vi "FW102C Engine.vi"(0 "Notifier Name":string="Not a Name", 11 "COM Port":string[](array[string])) -> ()   [LabVIEW 2016]
uses:
  FW Type Defs/FW Notifier Type.ctl
  FW Type Defs/FW Actions.ctl
  FilterWheel102_win64.dll
panel:
  out "FW ID":string
  out "Current Position":u8
  in  "Get Position":bool
  in  "FW Position":u8
  in  "Quit":bool
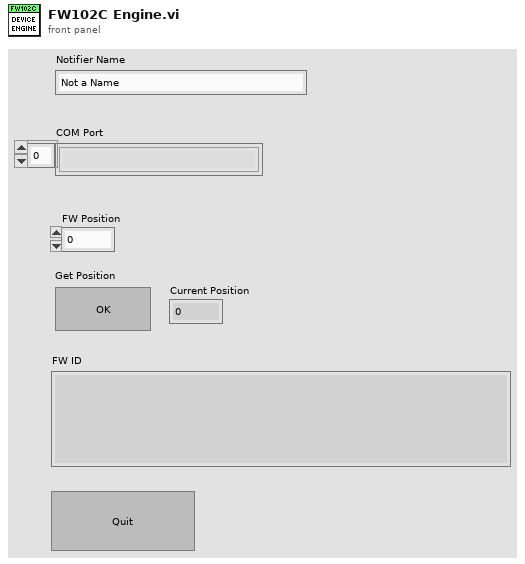
[diagram p1: front panel]
types:
  T1 = typedef "FW Actions.ctl" = enum16{"Set Position", "Get Position", "Get Num Positions", "Set Speed", "Quit"}
  T2 = typedef "FW Notifier Type.ctl" = cluster{"Actions":T1, "Set Position":u8, "Actual Position":u8, "Speed":dbl, "Num Positions":u8, "Received":bool}
  T3 = enum32{"Invalid", "Standard", "Closed", "Hidden", "Minimized", "Maximized"}
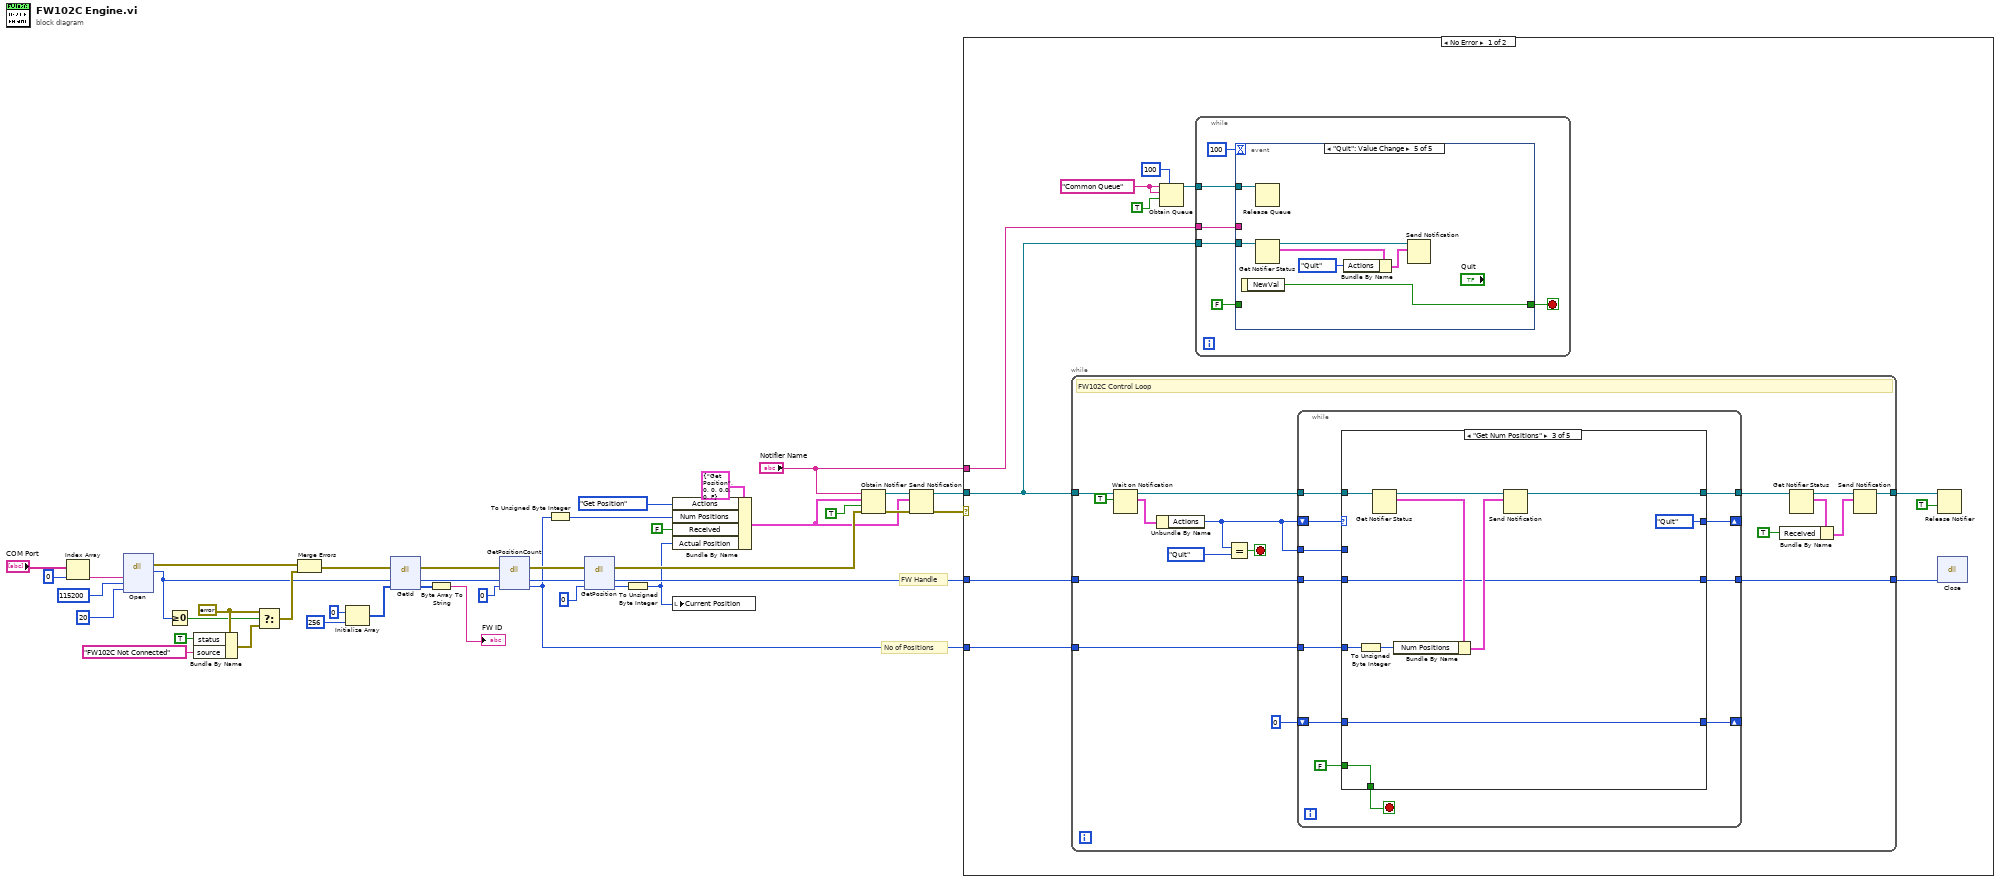
[diagram p0: block diagram]
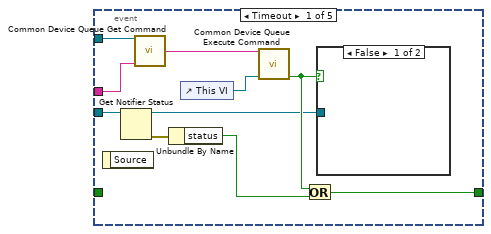
[diagram p2: hidden frame]
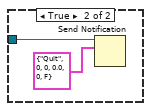
[diagram p3: hidden frame]
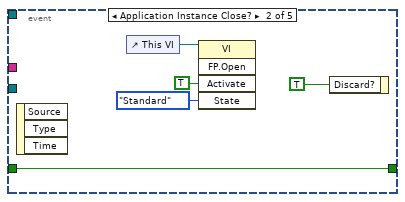
[diagram p4: hidden frame]
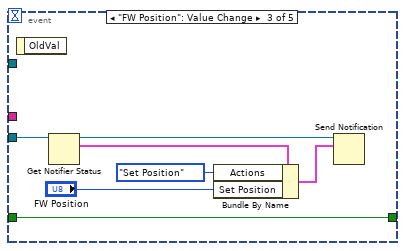
[diagram p5: hidden frame]
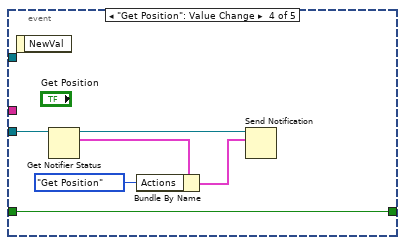
[diagram p6: hidden frame]
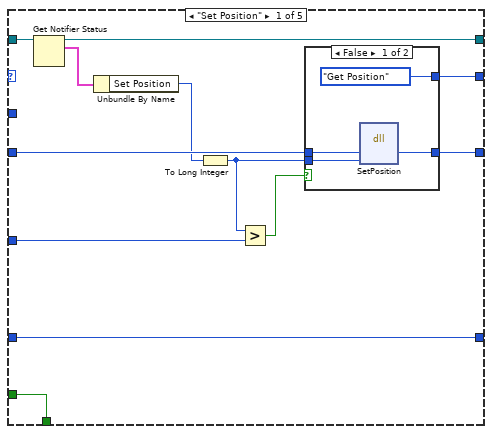
[diagram p7: hidden frame]
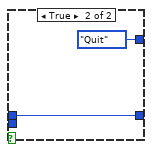
[diagram p8: hidden frame]
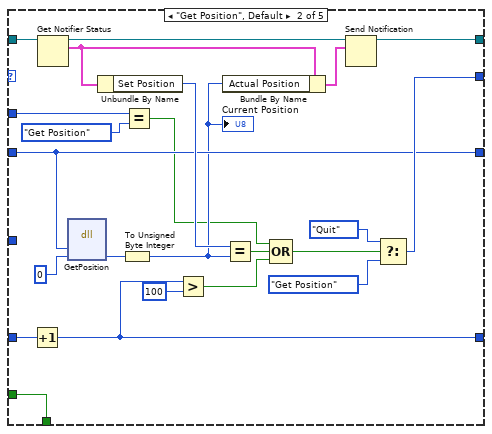
[diagram p9: hidden frame]
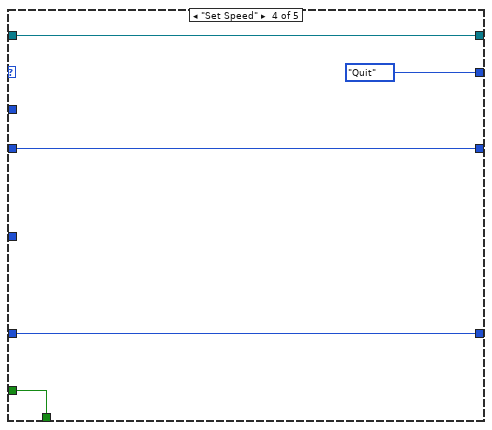
[diagram p10: hidden frame]
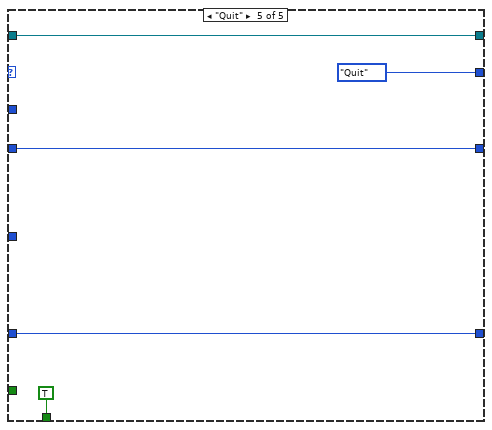
[diagram p11: hidden frame]
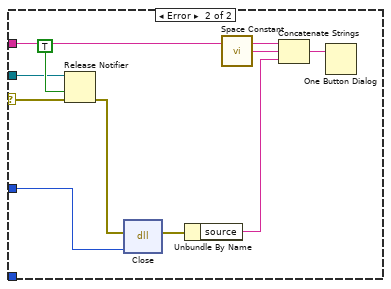
[diagram p12: hidden frame]
diagram:
  w30 = errorcluster {"status"=FALSE, "code"=0, "source"=""} ("error out")
  # "No of Positions"
  # "FW Handle"
  n1 = Index Array(array="COM Port", index=0) -> (element=w31:string)
  n2 = dll-call lib="C:/Users/gs519/Documents/Microscope-Control/Device Library/Filter Wheels/Thorlabs/FW102C/FilterWheel102_win64.dll" fn="Open"("Serial No"=w31, "nBaud"=115200 ("nbaud"), "timeout"=20) -> (error out=w25:errorcluster, "hdl"=w18:i32)  [unwired: 6 in, 1 out]
  n3 = Greater Or Equal To 0?(x=w18) -> (x >= 0?=w26:bool)
  n4 = Bundle By Name(cluster=w30, "status"=TRUE, "source"="FW102C Not Connected") -> (w27:errorcluster)
  n5 = Select(t=w30, s=w26, f=w27) -> (s? t:f=w24:errorcluster)
  n6 = Merge Errors(w25, w24) -> (w17:errorcluster)
  n7 = Initialize Array(u8 0 ("element"), 256 ("dimension size")) -> (w21:u8[])
  n8 = dll-call lib="C:/Users/gs519/Documents/Microscope-Control/Device Library/Filter Wheels/Thorlabs/FW102C/FilterWheel102_win64.dll" fn="GetId"(error in=w17, "hdl"=w18, "id"=w21) -> (error out=w15:errorcluster, "hdl"=w14:i32, "id"=w19:u8[])  [unwired: 3 in, 1 out]
  n9 = Byte Array To String(unsigned byte array=w19) -> (string=→"FW ID":string)
  n10 = dll-call lib="C:/Users/gs519/Documents/Microscope-Control/Device Library/Filter Wheels/Thorlabs/FW102C/FilterWheel102_win64.dll" fn="GetPositionCount" label="GetCount"(error in=w15, "hdl"=w14, "position count"=0) -> (error out=w12:errorcluster, "hdl"=w11:i32, "position count"=w2:i32)  [unwired: 3 in, 1 out]
  n11 = To Unsigned Byte Integer(number=w2) -> (unsigned 8bit integer=w1:u8)
  n12 = dll-call lib="C:/Users/gs519/Documents/Microscope-Control/Device Library/Filter Wheels/Thorlabs/FW102C/FilterWheel102_win64.dll" fn="GetPosition"(error in=w12, "hdl"=w11, "position"=0) -> (error out=w10:errorcluster, "hdl"=w9:i32, "position"=w5:i32)  [unwired: 3 in, 1 out]
  n13 = To Unsigned Byte Integer(number=w5) -> (unsigned 8bit integer=w3:u8)
  n14 = Bundle By Name(cluster=T2 {"Actions"=enum."Get Position", "Set Position"=0, "Actual Position"=0, "Speed"=0.0, "Num Positions"=0, "Received"=FALSE} ("Note Type"), "Actions"=FW_Actions."Get Position", "Num Positions"=w1, "Received"=FALSE ("Received?"), "Actual Position"=w3) -> (w4:T2)
  n15 = local write "Current Position"(w3) -> ()
  n16 = Obtain Notifier(name (unnamed)="Notifier Name", notification data type=w4, create if not found? (T)=TRUE, error in (no error)=w10) -> (notifier out=w40:refnum<notifier>, error out=w39:errorcluster)  [unwired: 1 out]
  n17 = Send Notification(notification=w4, notifier=w40, error in (no error)=w39) -> (notifier out=w38:refnum<notifier>, error out=w37:errorcluster)
  n18 = case shown="No Error" w37 {
    selector: w37 -> [_ w194]
    tunnel: w38 -> [w50 w195]
    tunnel: "Notifier Name" -> [w49 w193]
    tunnel: w9 -> [w44 w190]
    tunnel: w2 -> [w42 _]
    frame No Error {
      w48 = "Common Queue" ("Unique Notifier Name")
      n19 = while {
        tunnel: w50 -> [w106]
        tunnel: [w107] -> w51
        tunnel: w44 -> [w102]
        tunnel: [w101] -> w43
        tunnel: w42 -> [w100]
        stop <- w112 stop-if-true
        # "FW102C Control Loop"
        n20 = Wait on Notification(notifier=w106, ignore previous (F)=TRUE) -> (notifier out=w104:refnum<notifier>, notification=w99:T2)  [unwired: 2 in, 2 out]
        n21 = Unbundle By Name(w99) -> ("Actions"=w97:T1)
        n22 = Equal?(x=w97, y=FW_Actions."Quit") -> (x = y?=w112:bool)
        n23 = while {
          tunnel: w104 -> [w123]
          tunnel: [w122] -> w103
          tunnel: w102 -> [w119]
          tunnel: [w118] -> w101
          tunnel: w100 -> [w117]
          shift-right: [w115] -> _
          shift-left: u16 0 -> [w116]
          shift-right: [w114] -> _
          shift-left: w97 -> [w124]
          tunnel: w97 -> [w113]
          stop <- w120 stop-if-true
          n24 = case shown="\"Get Num Positions\"" w124 {
            tunnel: w123 -> [w131 w162 w175 w181 w186]
            tunnel: [w130 w160 w173 w181 w186] -> w122
            tunnel: [w136 w165 w176 w179 TRUE] -> w120
            tunnel: FALSE -> [w136 w165 w176 w179 _]
            tunnel: w119 -> [w133 w150 w167 w177 w184]
            tunnel: [w129 w150 w167 w177 w184] -> w118
            tunnel: w117 -> [w126 _ w170 _ _]
            tunnel: w116 -> [w135 w156 w166 w178 w183]
            tunnel: [w135 w152 w166 w178 w183] -> w115
            tunnel: [w134 w151 FW_Actions."Quit" ("f") FW_Actions."Quit" ("f") FW_Actions."Quit" ("f")] -> w114
            tunnel: w113 -> [_ w148 _ _ _]
            frame "Set Position" {
              n25 = Get Notifier Status(notifier=w131) -> (notifier out=w130:refnum<notifier>, current notification=w132:T2)  [unwired: 1 in, 3 out]
              n26 = Unbundle By Name(w132) -> ("Set Position"=w128:u8)
              n27 = To Long Integer(number=w128) -> (32bit integer=w127:i32)
              n28 = Greater?(x=w127, y=w126) -> (0:w125:bool)
              n29 = case shown="False" w125 {
                tunnel: [FW_Actions."Get Position" ("f") FW_Actions."Quit" ("f")] -> w134
                tunnel: w133 -> [w139 w142]
                tunnel: [w138 w142] -> w129
                tunnel: w127 -> [w137 _]
                frame False {
                  n30 = dll-call lib="C:/Users/gs519/Documents/Microscope-Control/Device Library/Filter Wheels/Thorlabs/FW102C/FilterWheel102_win64.dll" fn="SetPosition"("hdl"=w139, "position"=w137) -> ("hdl"=w138:i32)  [unwired: 5 in, 2 out]
                }
                frame True {
                }
              }
            }
            frame "Get Position", Default {
              n31 = Increment(x=w156) -> (x+1=w152:u16)
              n32 = Get Notifier Status(notifier=w162) -> (notifier out=w161:refnum<notifier>, current notification=w159:T2)  [unwired: 1 in, 3 out]
              n33 = dll-call lib="C:/Users/gs519/Documents/Microscope-Control/Device Library/Filter Wheels/Thorlabs/FW102C/FilterWheel102_win64.dll" fn="GetPosition"("hdl"=w150, "position"=0) -> ("position"=w164:i32)  [unwired: 5 in, 2 out]
              n34 = Unbundle By Name(w159) -> ("Set Position"=w157:u8)
              n35 = To Unsigned Byte Integer(number=w164) -> (unsigned 8bit integer=w149:u8)
              "Current Position" <- w149
              n36 = Equal?(x=w148, y=FW_Actions."Get Position") -> (x = y?=w144:bool)
              n37 = Greater?(x=w152, y=u16 100) -> (0:w145:bool)
              n38 = Bundle By Name(cluster=w159, "Actual Position"=w149) -> (w158:T2)
              n39 = Equal?(x=w157, y=w149) -> (x = y?=w146:bool)
              n40 = Compound Arithmetic op=OR(w144, w146, w145) -> (w143:bool)
              n41 = Send Notification(notification=w158, notifier=w161) -> (notifier out=w160:refnum<notifier>)  [unwired: 1 in, 1 out]
              n42 = Select(t=FW_Actions."Quit" ("y"), s=w143, f=FW_Actions."Get Position") -> (s? t:f=w151:T1)
            }
            frame "Get Num Positions" {
              n43 = To Unsigned Byte Integer(number=w170) -> (unsigned 8bit integer=w169:u8)
              n44 = Get Notifier Status(notifier=w175) -> (notifier out=w174:refnum<notifier>, current notification=w171:T2)  [unwired: 1 in, 3 out]
              n45 = Bundle By Name(cluster=w171, "Num Positions"=w169) -> (w168:T2)
              n46 = Send Notification(notification=w168, notifier=w174) -> (notifier out=w173:refnum<notifier>)  [unwired: 1 in, 1 out]
            }
            frame "Set Speed" {
            }
            frame "Quit" {
            }
          }
        }
        n47 = Get Notifier Status(notifier=w103) -> (notifier out=w108:refnum<notifier>, current notification=w110:T2)  [unwired: 1 in, 3 out]
        n48 = Bundle By Name(cluster=w110, "Received"=TRUE ("Received?")) -> (w111:T2)
        n49 = Send Notification(notification=w111, notifier=w108) -> (notifier out=w107:refnum<notifier>)  [unwired: 1 in, 1 out]
      }
      n50 = Obtain Queue(max queue size (-1, unlimited)=100, name (unnamed)=w48, element data type=w48, create if not found? (T)=TRUE) -> (queue out=w45:refnum<queue>)  [unwired: 1 in, 2 out]
      n51 = while {
        tunnel: w45 -> [w58]
        tunnel: w50 -> [w55]
        tunnel: w49 -> [w53]
        stop <- w54 stop-if-true
        n52 = event shown="[4] \"Quit\": Value Change" {
          selector: _ -> [_ _ _ _ _]
          dyn-events: _ -> [_ _ _ _ _]
          timeout: 100 -> [_ _ _ _ _]
          tunnel: w58 -> [w66 _ _ _ w91]
          tunnel: FALSE -> [_ w75 w82 w88 _]
          tunnel: w55 -> [w68 _ w81 w87 w92]
          tunnel: [w61 w75 w82 w88 w95] -> w54
          tunnel: w53 -> [w65 _ _ _ _]
          event Timeout {
            n53 = event-data() -> ()  [unwired: 1 in, 1 out]
            n54 = Get Notifier Status(notifier=w68) -> (notifier out=w59:refnum<notifier>, error out=w67:errorcluster)  [unwired: 1 in, 3 out]
            n55 = call "Common Device Queue Get Command.vi"("Common Queue"=w66, "Notifier Name"=w65) -> ("Command"=w64:string)  [unwired: 12 in, 1 out]
            n56 = Unbundle By Name(w67) -> ("status"=w62:bool)
            n57 = control-ref of="This VI"() -> (w63:refnum<vi>)
            n58 = call "Common Device Queue Execute Command.vi"("Common Command"=w64, "VI Refnum"=w63) -> ("Quit?"=w60:bool)  [unwired: 12 in, 1 out]
            n59 = Or(x=w60, y=w62) -> (x .or. y?=w61:bool)
            n60 = case shown="False" w60 {
              tunnel: w59 -> [_ w70]
              frame False {
              }
              frame True {
                n61 = Send Notification(notification=T2 {"Actions"=enum."Quit", "Set Position"=0, "Actual Position"=0, "Speed"=0.0, "Num Positions"=0, "Received"=FALSE} ("Note Type"), notifier=w70) -> ()  [unwired: 1 in, 2 out]
              }
            }
          }
          event Application Instance Close? {
            n62 = event-data() -> ()  [unwired: 1 in, 3 out]
            n63 = control-ref of="This VI"() -> (w72:refnum<vi>)
            n64 = invoke class="VI" method="FP.Open"(reference=w72, "Activate"=TRUE ("Activate?"), "State"=T3."Standard") -> ()  [unwired: 2 in, 5 out]
            n65 = event-data("Discard?"=TRUE) -> ()  [unwired: 1 in, 1 out]
          }
          event "FW Position": Value Change {
            n66 = event-data() -> ()  [unwired: 1 in, 1 out]
            n67 = Get Notifier Status(notifier=w81) -> (notifier out=w80:refnum<notifier>, current notification=w79:T2)  [unwired: 1 in, 3 out]
            n68 = Bundle By Name(cluster=w79, "Actions"=FW_Actions."Set Position", "Set Position"="FW Position") -> (w78:T2)
            n69 = Send Notification(notification=w78, notifier=w80) -> ()  [unwired: 1 in, 2 out]
          }
          event "Get Position": Value Change {
            n70 = event-data() -> ()  [unwired: 1 in, 1 out]
            n71 = Get Notifier Status(notifier=w87) -> (notifier out=w86:refnum<notifier>, current notification=w85:T2)  [unwired: 1 in, 3 out]
            n72 = Bundle By Name(cluster=w85, "Actions"=FW_Actions."Get Position") -> (w84:T2)
            n73 = Send Notification(notification=w84, notifier=w86) -> ()  [unwired: 1 in, 2 out]
          }
          event "Quit": Value Change {
            n74 = event-data() -> ("NewVal"=w95:bool)  [unwired: 1 in]
            n75 = Release Queue(queue=w91) -> ()  [unwired: 2 in, 3 out]
            n76 = Get Notifier Status(notifier=w92) -> (notifier out=w94:refnum<notifier>, current notification=w90:T2)  [unwired: 1 in, 3 out]
            n77 = Bundle By Name(cluster=w90, "Actions"=FW_Actions."Quit") -> (w93:T2)
            n78 = Send Notification(notification=w93, notifier=w94) -> ()  [unwired: 1 in, 2 out]
          }
        }
      }
      n79 = Release Notifier(notifier=w51, force destroy? (F)=TRUE) -> ()  [unwired: 1 in, 3 out]
      n80 = dll-call lib="C:/Users/gs519/Documents/Microscope-Control/Device Library/Filter Wheels/Thorlabs/FW102C/FilterWheel102_win64.dll" fn="Close"("hdl"=w43) -> ()  [unwired: 5 in, 2 out]
    }
    frame Error {
      n81 = Release Notifier(notifier=w195, force destroy? (F)=TRUE, error in (no error)=w194) -> (error out=w189:errorcluster)  [unwired: 2 out]
      n82 = dll-call lib="C:/Users/gs519/Documents/Microscope-Control/Device Library/Filter Wheels/Thorlabs/FW102C/FilterWheel102_win64.dll" fn="Close"(error in=w189, "hdl"=w190) -> (error out=w188:errorcluster)  [unwired: 4 in, 1 out]
      n83 = Unbundle By Name(w188) -> ("source"=w187:string)
      n84 = call <vilib>:"Space Constant.vi"() -> ("String"=w191:string)
      n85 = Concatenate Strings(w193, w191, w187) -> (w192:string)
      n86 = One Button Dialog(message=w192) -> ()  [unwired: 1 in, 1 out]
    }
  }
